vi "Digitizer Scan Fetch Power.vi"(0 "instrument handle":refnum<k15>, 1 "LastPoint":i32 format="%.0g", 2 "CurrentChannel":string, 5 "Scale":dbl, 7 "Record":i32 format="%.0g", 9 "FirstPoint":i32 format="%.0g", 11 "error in (no error)":errorcluster {"code" format="%.0x"}, 12 "VoltageChannel":string, 13 "ValBufferSize":i32=2048) -> (4 "instrument handle out":refnum<k15>, 6 "Val":dbl[](array[numeric]) format="%.2p", 8 "ValActualSize":i32, 15 "error out":errorcluster {"code" format="%.0x"})   [LabVIEW 2020, in "Keysight DAQ970.lvlib"]
doc: "Performs post-processing calculation on the specified range of readings and returns power on the specified record for a paired/ coupled channel."
uses:
  Keysight DAQ970.lvlib
  KtDAQ970.dll
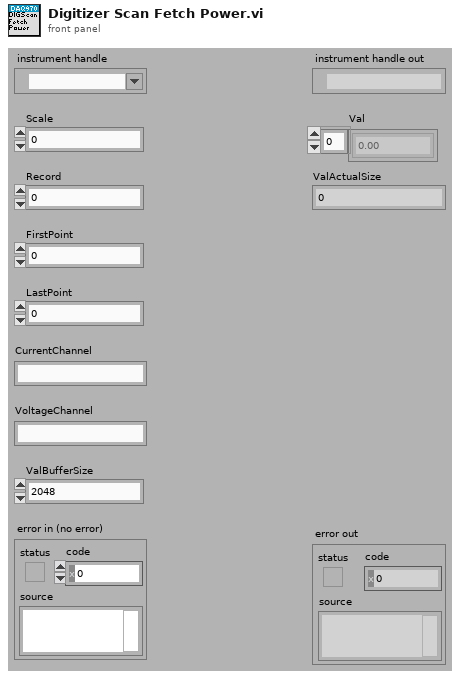
[diagram p1: front panel]
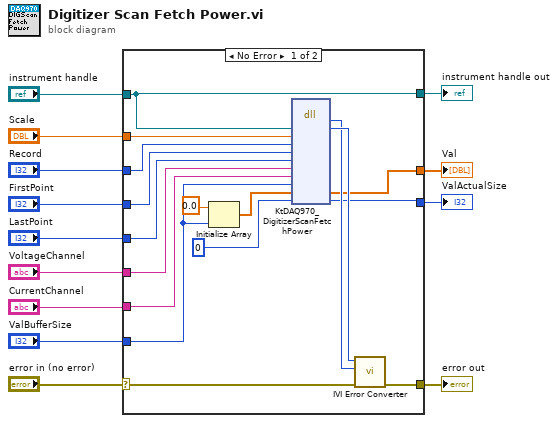
[diagram p0: block diagram]
diagram:
  n1 = case shown="No Error" "error in (no error)" {
    selector: "error in (no error)" -> [w28 w32]
    tunnel: [w27 w32] -> w13
    tunnel: "instrument handle" -> [w15 w31]
    tunnel: "Scale" -> [w26 _]
    tunnel: "Record" -> [w25 _]
    tunnel: "FirstPoint" -> [w24 _]
    tunnel: "LastPoint" -> [w23 _]
    tunnel: "VoltageChannel" -> [w22 _]
    tunnel: "CurrentChannel" -> [w21 _]
    tunnel: "ValBufferSize" -> [w14 _]
    tunnel: [w18 _] -> w3
    tunnel: [w16 _] -> w2
    tunnel: [w15 w31] -> w1
    frame No Error {
      n2 = Initialize Array(0.0 ("element"), w14) -> (w20:dbl[])
      n3 = dll-call lib="KtDAQ970**.dll" fn="KtDAQ970_DigitizerScanFetchPower"("Vi"=w15, "Scale"=w26, "Record"=w25, "FirstPoint"=w24, "LastPoint"=w23, "VoltageChannel"=w22, "CurrentChannel"=w21, "ValBufferSize"=w14, "Val"=w20, "ValActualSize"=0) -> (w29:i32, "Vi"=w30:u32, "Val"=w18:dbl[], "ValActualSize"=w16:i32)  [unwired: 10 in, 2 out]
      n4 = call "IVI Error Converter.vi"("error in (no error)"=w28, "IVI error code (0)"=w29, "instrument handle"=w30) -> ("error out"=w27:errorcluster)  [unwired: 7 in, 1 out]
    }
    frame Error {
    }
  }
  "error out" <- w13
  "instrument handle out" <- w1
  "Val" <- w3
  "ValActualSize" <- w2
